vi "Moving Average Filter.vi"(8 "error in (no error)":errorcluster, 11 "Values":dbl[](array[numeric])) -> (0 "error out":errorcluster, 1 "Count":i32, 2 "Averaged Values":dbl[](array[numeric]), 3 "Buffer":dbl[][](array[numeric]))   [LabVIEW 2015]
doc: "This VI implements a moving average filter for this particular channel"
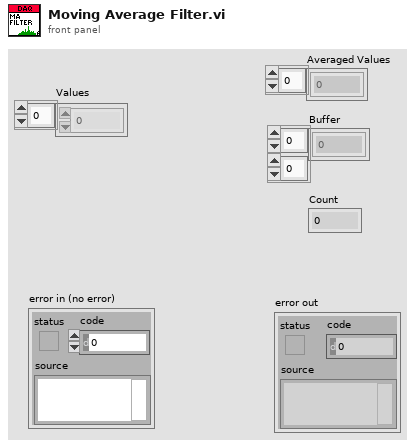
[diagram p1: front panel]
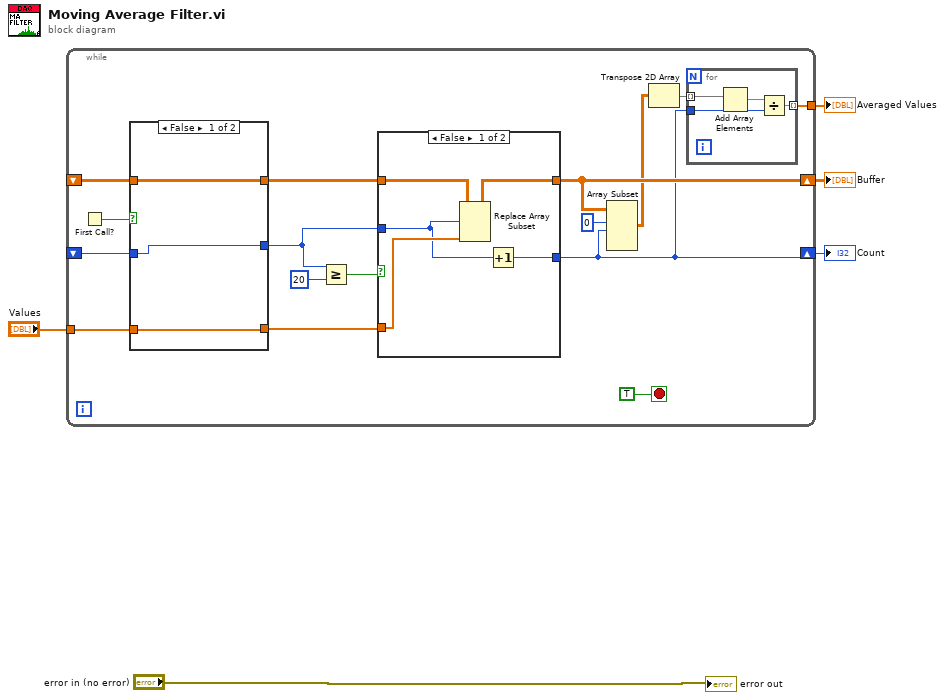
[diagram p0: block diagram]
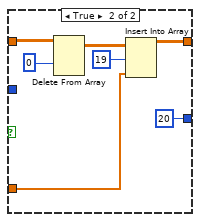
[diagram p2: hidden frame]
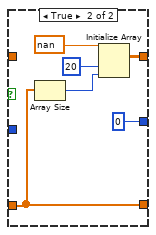
[diagram p3: hidden frame]
diagram:
  n1 = while {
    tunnel: "Values" -> [w12]
    shift-right: [w16] -> w2
    shift-left: _ -> [w15]
    shift-right: [w8] -> w1
    shift-left: _ -> [w14]
    tunnel: [w7] -> w3
    stop <- TRUE stop-if-true
    n2 = First Call?() -> (First Call?: T/F=w21:bool)
    n3 = case shown="False" w21 {
      tunnel: [w40 w45] -> w13
      tunnel: [w39 0 ("dimension size")] -> w18
      tunnel: w15 -> [w40 _]
      tunnel: w14 -> [w39 _]
      tunnel: w12 -> [w38 w43]
      tunnel: [w38 w43] -> w11
      frame False {
      }
      frame True {
        n4 = Array Size(array=w43) -> (size(s)=w41:i32)
        n5 = Initialize Array(nan ("element"), 20 ("dimension size"), w41) -> (w45:dbl[][])
      }
    }
    n6 = Greater Or Equal?(x=w18, y=20) -> (x >= y?=w19:bool)
    n7 = case shown="False" w19 {
      tunnel: w13 -> [w30 w37]
      tunnel: w18 -> [w26 _]
      tunnel: [w29 w35] -> w16
      tunnel: [w28 20] -> w8
      tunnel: w11 -> [w27 w33]
      frame False {
        n8 = Replace Array Subset(array=w30, new element=w27, index (row)=w26) -> (w29:dbl[][])  [unwired: 1 in]
        n9 = Increment(x=w26) -> (x+1=w28:i32)
      }
      frame True {
        n10 = Delete From Array(array=w37, index (row)=0 ("index")) -> (array with subset deleted=w36:dbl[][])  [unwired: 2 in, 1 out]
        n11 = Insert Into Array(array=w36, index (row)=19 ("index"), new element=w33) -> (w35:dbl[][])  [unwired: 1 in]
      }
    }
    n12 = Array Subset(array=w16, index (row)=0 ("index"), length (row)=w8) -> (w9:dbl[][])  [unwired: 2 in]
    n13 = Transpose 2D Array(2D array=w9) -> (transposed array=w6:dbl[][])
    n14 = for {
      tunnel: w6 -> [w25] mode=indexing
      tunnel: w8 -> [w23]
      tunnel: [w22] -> w7 mode=indexing
      n15 = Add Array Elements(numeric array=w25) -> (sum=w24:dbl)
      n16 = Divide(x=w24, y=w23) -> (x/y=w22:dbl)
    }
  }
  "Averaged Values" <- w3
  "Buffer" <- w2
  "Count" <- w1
  "error out" <- "error in (no error)"
